vi "lab2.vi"() -> ()   [LabVIEW 2019]
uses:
  <vilib>/imath/engines/lvmath2/RunTimeEngine/BuiltInFunctions/iir_elliptic/NIMS_[2o]_iir_elliptic(I32,DBL2,V,Str).vi
  <vilib>/imath/engines/lvmath2/RunTimeEngine/ErrorHandling/NIMS_Create Error From Enums.vi
  <vilib>/imath/engines/lvmath/Plug In/Control Design/BuiltInFunctions/tf/NIMS_CD_tf(num,den,Ts).vi
  <vilib>/imath/engines/lvmath2/RunTimeEngine/BuiltInFunctions/iir_elliptic/NIMS_[3o]_iir_elliptic(I32,DBL2,V,Str).vi
  <vilib>/imath/engines/lvmath/Plug In/Control Design/BuiltInFunctions/zpk/NIMS_CD_zpk(zeros,poles,k,Ts).vi
  <vilib>/imathl/engines/lvmath/Functions/Error Handling/Create Error.vi
  <vilib>/imath/engines/lvmath2/RunTimeEngine/BuiltInFunctions/iir_elliptic/NIMS_[4o]_iir_elliptic(I32,DBL2,V,Str).vi
  <vilib>/imath/engines/lvmath/Plug In/Control Design/BuiltInFunctions/ss/NIMS_CD_ss(A,B,C,D).vi
  <vilib>/imath/engines/lvmath2/RunTimeEngine/NodeEndStatement/NIMS_NodeEndStatement_Output.vi
  <instcachedir>/0/NIMS_NodeEndStatement_Output_53EC0D466D134D7ABD903AC30B43404B.lvgen/NIMS_NodeEndStatement_Output_53EC0D466D134D7ABD903AC30B43404B_011.vi
  <instcachedir>/0/NIMS_NodeEndStatement_Output_53EC0D466D134D7ABD903AC30B43404B.lvgen/NIMS_NodeEndStatement_Output_53EC0D466D134D7ABD903AC30B43404B_010.vi
  <instcachedir>/0/NIMS_NodeEndStatement_Output_53EC0D466D134D7ABD903AC30B43404B.lvgen/NIMS_NodeEndStatement_Output_53EC0D466D134D7ABD903AC30B43404B_009.vi
  <vilib>/imath/engines/lvmath2/RunTimeEngine/ErrorHandling/NIMS_Finalize Error.vi
  <vilib>/addons/Control Design/_Utility/Model Viewer.llb/Model Viewer SubVI/cd_Draw State-Space Equation (SS).vi
  <vilib>/addons/Control Design/_Utility/Model Viewer.llb/Model Viewer SubVI/cd_Draw Zero-Pole-Gain Equation (ZPK).vi
  <vilib>/addons/Control Design/_Utility/Model Viewer.llb/Model Viewer SubVI/cd_Draw Transfer Function Equation (TF).vi
  <vilib>/addons/Control Design/_Time Response Analysis/Time Response.llb/Time Response subVI/cd_Step Response (Transfer Function).vi
  <vilib>/addons/Control Design/_Time Response Analysis/Time Response.llb/Time Response subVI/cd_Step Response (Zero-Pole-Gain).vi
  <vilib>/addons/Control Design/_Time Response Analysis/Time Response.llb/Time Response subVI/cd_Step Response (State-Space).vi
  <vilib>/addons/Control Design/_Utility/NI_CD_Model Viewer.lvlib
  <vilib>/addons/Control Design/_Time Response Analysis/NI_CD_Time Response.lvlib
panel:
  out "Нули, полюса и коэффициент усиления (zpk)":picture
  out "Реакция на ступенчатое воздействие":cluster{"time":dbl[], dbl[]}[](graph)
  out "Погрешность реакции на ступенчатое воздействие":cluster{"time":dbl[], dbl[]}[](graph)
  out "Передаточная функция":picture
  out "Модель в пространстве состояний":picture
  in  "dbp":dbl
  in  "n":dbl
  in  "dbs":dbl
  in  "w":dbl
  in  "Time Range":cluster{"t0":dbl, "dt":dbl, "tf":dbl}
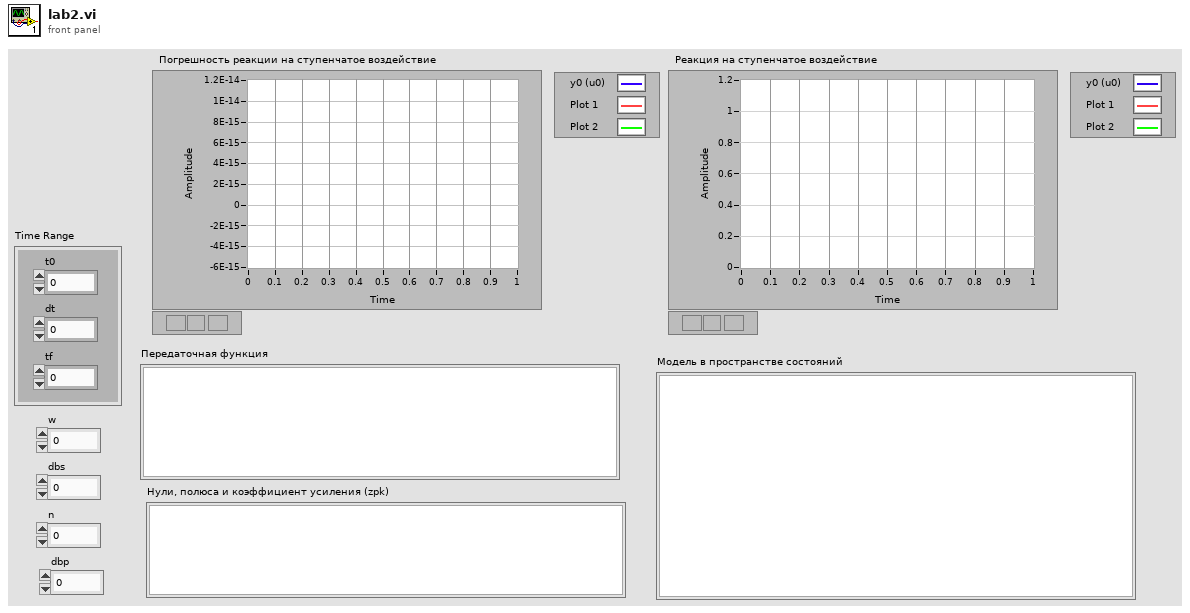
[diagram p1: front panel]
types:
  T1 = typedef "NI_LinSys_Model Typedefs.lvlib/CD Transfer Function Model (MIMO).ctl" = cluster{"properties":T2, "transfer function(s)":T3[][]}
  T2 = typedef "NI_LinSys_Model Typedefs.lvlib/CD General Elements.ctl" = cluster{"Model name":string, "Input names":string[], "Output names":string[], "Input Delays":dbl[], "Output Delays":dbl[], "Sampling Time":dbl, "Notes":string}
  T3 = typedef "NI_LinSys_Model Typedefs.lvlib/CD Transfer Function Model (SISO).ctl" = cluster{"Numerator":dbl[], "Denominator":dbl[], "delay":dbl}
  T4 = typedef "NI_LinSys_Model Typedefs.lvlib/CD Zero-Pole-Gain Model (MIMO).ctl" = cluster{"properties":T2, "zero-pole-gain(s)":T5[][]}
  T5 = typedef "NI_LinSys_Model Typedefs.lvlib/CD Zero-Pole-Gain Model (SISO).ctl" = cluster{"Gain":dbl, "Zeros":cdb[], "Poles":cdb[], "delay":dbl}
  T6 = typedef "NI_LinSys_Model Typedefs.lvlib/CD State Space Model (MIMO).ctl" = cluster{"properties":T2, "A":dbl[][], "B":dbl[][], "C":dbl[][], "D":dbl[][], "StateNames":string[], "Transport Delay":dbl[][]}
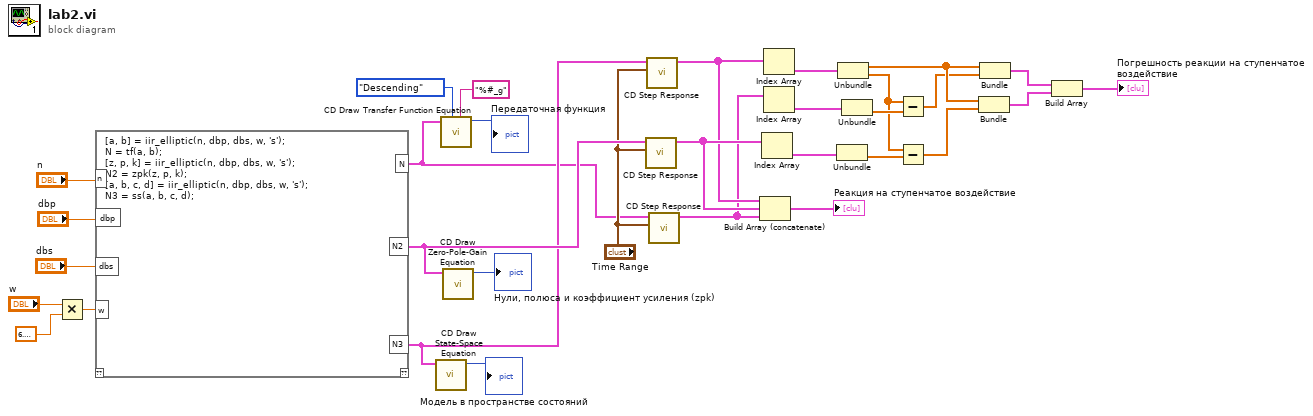
[diagram p0: block diagram]
diagram:
  n1 = Multiply(x="w", y=6.283185307179586) -> (x*y=w30:dbl)
  n2 = mathscript code="[a, b] = iir_elliptic(n, dbp, dbs, w, 's');\nN = tf(a, b);\n[z, p, k] = iir_elliptic(n, dbp, dbs, w, 's');\nN2 = zpk(z, p, k);\n[a, b, c, d] = iir_elliptic(n, dbp, dbs, w, 's');\nN3 = ss(a, b, c, d);"("n"="n", "dbp"="dbp", "dbs"="dbs", "w"=w30) -> ("N"=w18:T1, "N2"=w25:T4, "N3"=w19:T6)  [unwired: 1 in, 1 out]
  n3 = call-poly <vilib>:"CD Draw State-Space Equation.vi"("State-Space Model"=w19) -> ("Equation"=→"Модель в пространстве состояний":picture)  [unwired: 8 in, 2 out]
  n4 = call-poly <vilib>:"CD Draw Transfer Function Equation.vi"("Format Coefficients"="%#_g", "Display Format"=enum16{"", "Ascending", "Descending"}."Descending", "Transfer Function Model"=w18) -> ("Equation"=→"Передаточная функция":picture)  [unwired: 6 in, 2 out]
  n5 = call-poly <vilib>:"CD Draw Zero-Pole-Gain Equation.vi"("Zero-Pole-Gain Model"=w25) -> ("Equation"=→"Нули, полюса и коэффициент усиления (zpk)":picture)  [unwired: 8 in, 2 out]
  n6 = call-poly <vilib>:"CD Step Response.vi"("Time Range"="Time Range", "Zero-Pole-Gain Model"=w25) -> ("Step Response Graph"=w3:cluster{"time":dbl[], dbl[]}[])  [unwired: 7 in, 2 out]
  n7 = call-poly <vilib>:"CD Step Response.vi"("Time Range"="Time Range", "State-Space Model"=w19) -> ("Step Response Graph"=w2:cluster{"time":dbl[], dbl[]}[])  [unwired: 6 in, 3 out]
  n8 = call-poly <vilib>:"CD Step Response.vi"("Time Range"="Time Range", "Transfer Function Model"=w18) -> ("Step Response Graph"=w1:cluster{"time":dbl[], dbl[]}[])  [unwired: 7 in, 2 out]
  n9 = Build Array (concatenate)(w2, w3, w1) -> (→"Реакция на ступенчатое воздействие":cluster{"time":dbl[], dbl[]}[])
  n10 = Index Array(array=w3) -> (element=w15:cluster{"time":dbl[], dbl[]})  [unwired: 1 in]
  n11 = Index Array(array=w2) -> (element=w17:cluster{"time":dbl[], dbl[]})  [unwired: 1 in]
  n12 = Index Array(array=w1) -> (element=w16:cluster{"time":dbl[], dbl[]})  [unwired: 1 in]
  n13 = Unbundle(w15) -> (w12:dbl[])  [unwired: 1 out]
  n14 = Unbundle(w17) -> ("time"=w14:dbl[], w11:dbl[])
  n15 = Unbundle(w16) -> (w13:dbl[])  [unwired: 1 out]
  n16 = Subtract(x=w11, y=w13) -> (x-y=w10:dbl[])
  n17 = Subtract(x=w11, y=w12) -> (x-y=w9:dbl[])
  n18 = Bundle("time"=w14, w9) -> (w7:cluster{"time":dbl[], dbl[]})  [unwired: 1 in]
  n19 = Bundle("time"=w14, w10) -> (w8:cluster{"time":dbl[], dbl[]})  [unwired: 1 in]
  n20 = Build Array(w8, w7) -> (→"Погрешность реакции на ступенчатое воздействие":cluster{"time":dbl[], dbl[]}[])
